vi "25_2_cholesky_decomposition.vi"(1 "n":i32, 2 "m":i32, 3 "A":fxp<+/-,25,2>[](array[numeric])) -> (0 "L":fxp<+/-,25,2>[](array[numeric]))   [LabVIEW 2020]
panel:
  in  "s":fxp<+/-,25,2>
  in  "L_type":fxp<+/-,25,2>
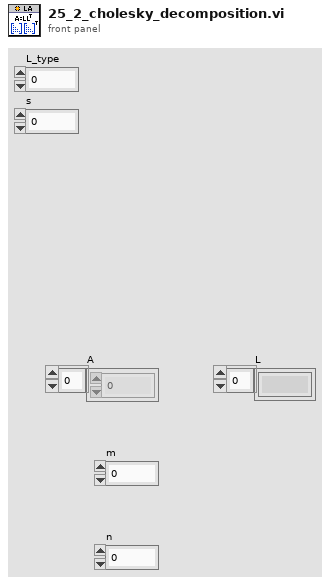
[diagram p1: front panel]
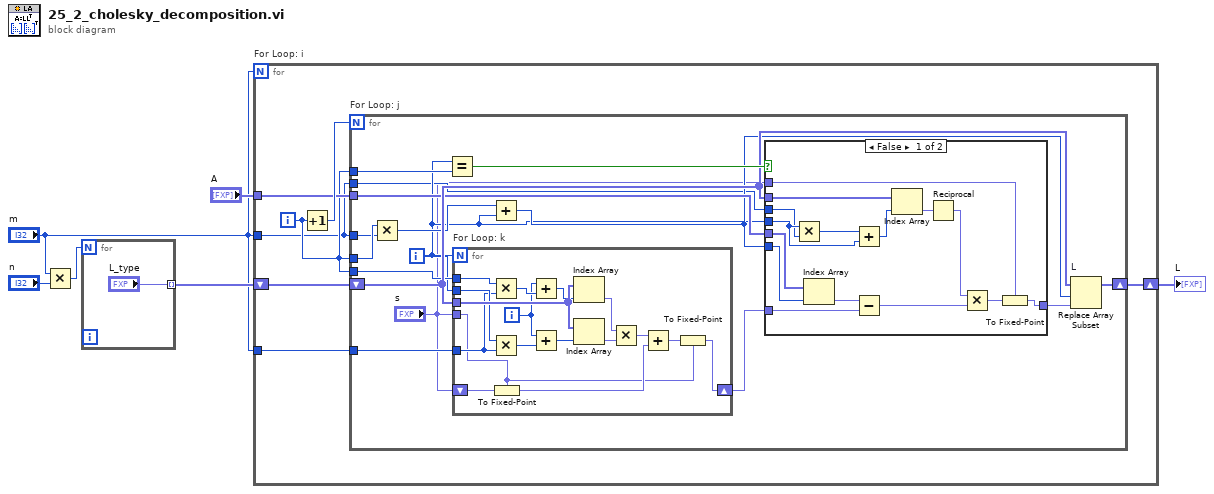
[diagram p0: block diagram]
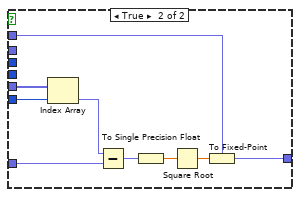
[diagram p2: hidden frame]
diagram:
  n1 = Multiply(x="m", y="n") -> (x*y=w1:i32)
  n2 = for {
    N: w1 -> [_]
    tunnel: ["L_type"] -> w4 mode=indexing
  }
  n3 = for "For Loop: i" {
    N: "m" -> [_]
    shift-right: [w12] -> w6
    shift-left: w4 -> [w14]
    tunnel: "A" -> [w11]
    tunnel: "m" -> [w9]
    tunnel: "m" -> [w8]
    i -> [w10]
    n4 = Increment(x=w10) -> (x+1=w13:i32)
    n5 = for "For Loop: j" {
      N: w13 -> [_]
      tunnel: w10 -> [w25]
      shift-right: [w27] -> w12
      shift-left: w14 -> [w26]
      tunnel: w10 -> [w24]
      tunnel: w11 -> [w22]
      tunnel: w10 -> [w20]
      tunnel: w9 -> [w18]
      tunnel: w9 -> [w17]
      tunnel: w8 -> [w16]
      i -> [w19]
      n6 = Multiply(x=w24, y=w18) -> (x*y=w23:i32)
      n7 = Equal?(x=w19, y=w25) -> (x = y?=w30:bool)
      n8 = for "For Loop: k" {
        N: w19 -> [_]
        tunnel: w26 -> [w71]
        shift-right: [w56] -> w29
        shift-left: "s" -> [w59]
        tunnel: w20 -> [w68]
        tunnel: w19 -> [w63]
        tunnel: w16 -> [w61]
        tunnel: "s" -> [w55]
        i -> [w62]
        n9 = Multiply(x=w68, y=w61) -> (x*y=w67:i32)
        n10 = Multiply(x=w63, y=w61) -> (x*y=w65:i32)
        n11 = To Fixed-Point(fixed-point type=w55, number=w59) -> (fixed-point=w58:fxp<+/-,25,2>)
        n12 = Add(x=w62, y=w67) -> (x+y=w66:i32)
        n13 = Add(x=w62, y=w65) -> (x+y=w64:i32)
        n14 = Index Array(array=w71, index=w66) -> (element=w60:fxp<+/-,25,2>)
        n15 = Index Array(array=w71, index=w64) -> (element=w70:fxp<+/-,25,2>)
        n16 = Multiply(x=w60, y=w70) -> (x*y=w69:fxp<+/-,50,4>)
        n17 = Add(x=w69, y=w58) -> (x+y=w57:fxp<+/-,50,4>)
        n18 = To Fixed-Point(fixed-point type=w55, number=w57) -> (fixed-point=w56:fxp<+/-,25,2>)
      }
      n19 = Add(x=w23, y=w19) -> (x+y=w21:i32)
      n20 = case shown="False" w30 {
        tunnel: w29 -> [w43 w54]
        tunnel: [w32 w47] -> w28
        tunnel: w26 -> [w45 _]
        tunnel: w22 -> [w40 w53]
        tunnel: w21 -> [w39 w52]
        tunnel: w19 -> [w36 _]
        tunnel: w17 -> [w34 _]
        tunnel: "s" -> [w31 w46]
        frame False {
          n21 = Multiply(x=w36, y=w34) -> (x*y=w37:i32)
          n22 = Index Array(array=w40, index=w39) -> (element=w38:fxp<+/-,25,2>)
          n23 = Add(x=w37, y=w36) -> (x+y=w35:i32)
          n24 = Subtract(x=w38, y=w43) -> (x-y=w41:fxp<+/-,26,3>)
          n25 = Index Array(array=w45, index=w35) -> (element=w44:fxp<+/-,25,2>)
          n26 = Reciprocal(x=w44) -> (1/x=w42:fxp<+/-,27,25>)
          n27 = Multiply(x=w42, y=w41) -> (x*y=w33:fxp<+/-,51,26>)
          n28 = To Fixed-Point(fixed-point type=w31, number=w33) -> (fixed-point=w32:fxp<+/-,25,2>)
        }
        frame True {
          n29 = Index Array(array=w53, index=w52) -> (element=w51:fxp<+/-,25,2>)
          n30 = Subtract(x=w51, y=w54) -> (x-y=w50:fxp<+/-,26,3>)
          n31 = To Single Precision Float(number=w50) -> (single precision float=w49:sgl)
          n32 = Square Root(x=w49) -> (sqrt(x)=w48:sgl)
          n33 = To Fixed-Point(fixed-point type=w46, number=w48) -> (fixed-point=w47:fxp<+/-,25,2>)
        }
      }
      n34 = Replace Array Subset "L"(array=w26, new element=w28, index=w21) -> (w27:fxp<+/-,25,2>[])
    }
  }
  "L" <- w6
